vi "cfcAPDtraj.vi"(0 "file path (use dialog)":path, 1 "Save Trajectory?":bool, 2 "Trajectory length (s)":dbl=5.0 format="%#_13g", 3 "FRET Refnum":refnum<vi>, 4 "Stop Refnum":refnum<vi>, 5 "error in (no error)":errorcluster) -> (6 "FRET Traj":cluster{i32, i32}(graph), 8 "error out":errorcluster)   [LabVIEW 2015]
uses:
  <vilib>/DAQmx/write.llb/DAQmx Write (Digital Bool 1Line 1Point).vi
  <vilib>/DAQmx/read.llb/DAQmx Read (Counter 1D U32 1Chan NSamp).vi
  <vilib>/DAQmx/create/channels.llb/DAQmx Create Channel (CI-Count Edges).vi
  <vilib>/DAQmx/configure/timing.llb/DAQmx Timing (Sample Clock).vi
  <vilib>/DAQmx/create/channels.llb/DAQmx Create Channel (CO-Pulse Generation-Time).vi
  <vilib>/DAQmx/configure/trigger.llb/DAQmx Start Trigger (Digital Edge).vi
  <vilib>/DAQmx/create/channels.llb/DAQmx Create Channel (DO-Digital Output).vi
  <vilib>/DAQmx/miscellaneous.llb/DAQmx Fill In Error Info.vi
  <resource>/objmgr/daqmx.rc
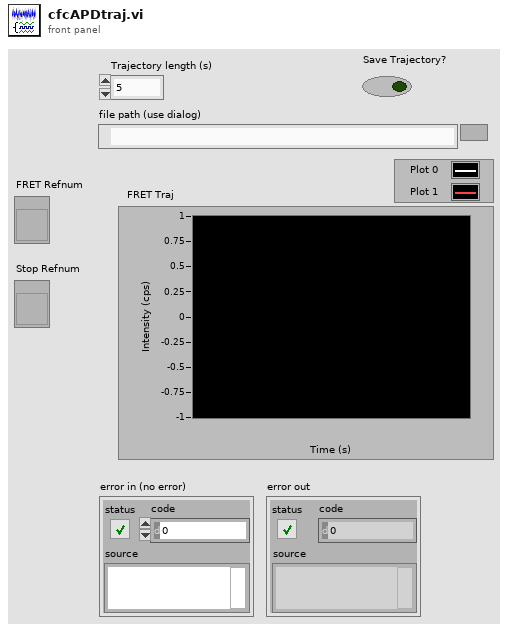
[diagram p1: front panel]
types:
  T1 = enum16{"big-endian, network order", "native, host order", "little-endian"}
  T2 = enum16{"open", "replace", "create", "open or create", "replace or create", "replace or create with confirmation"}
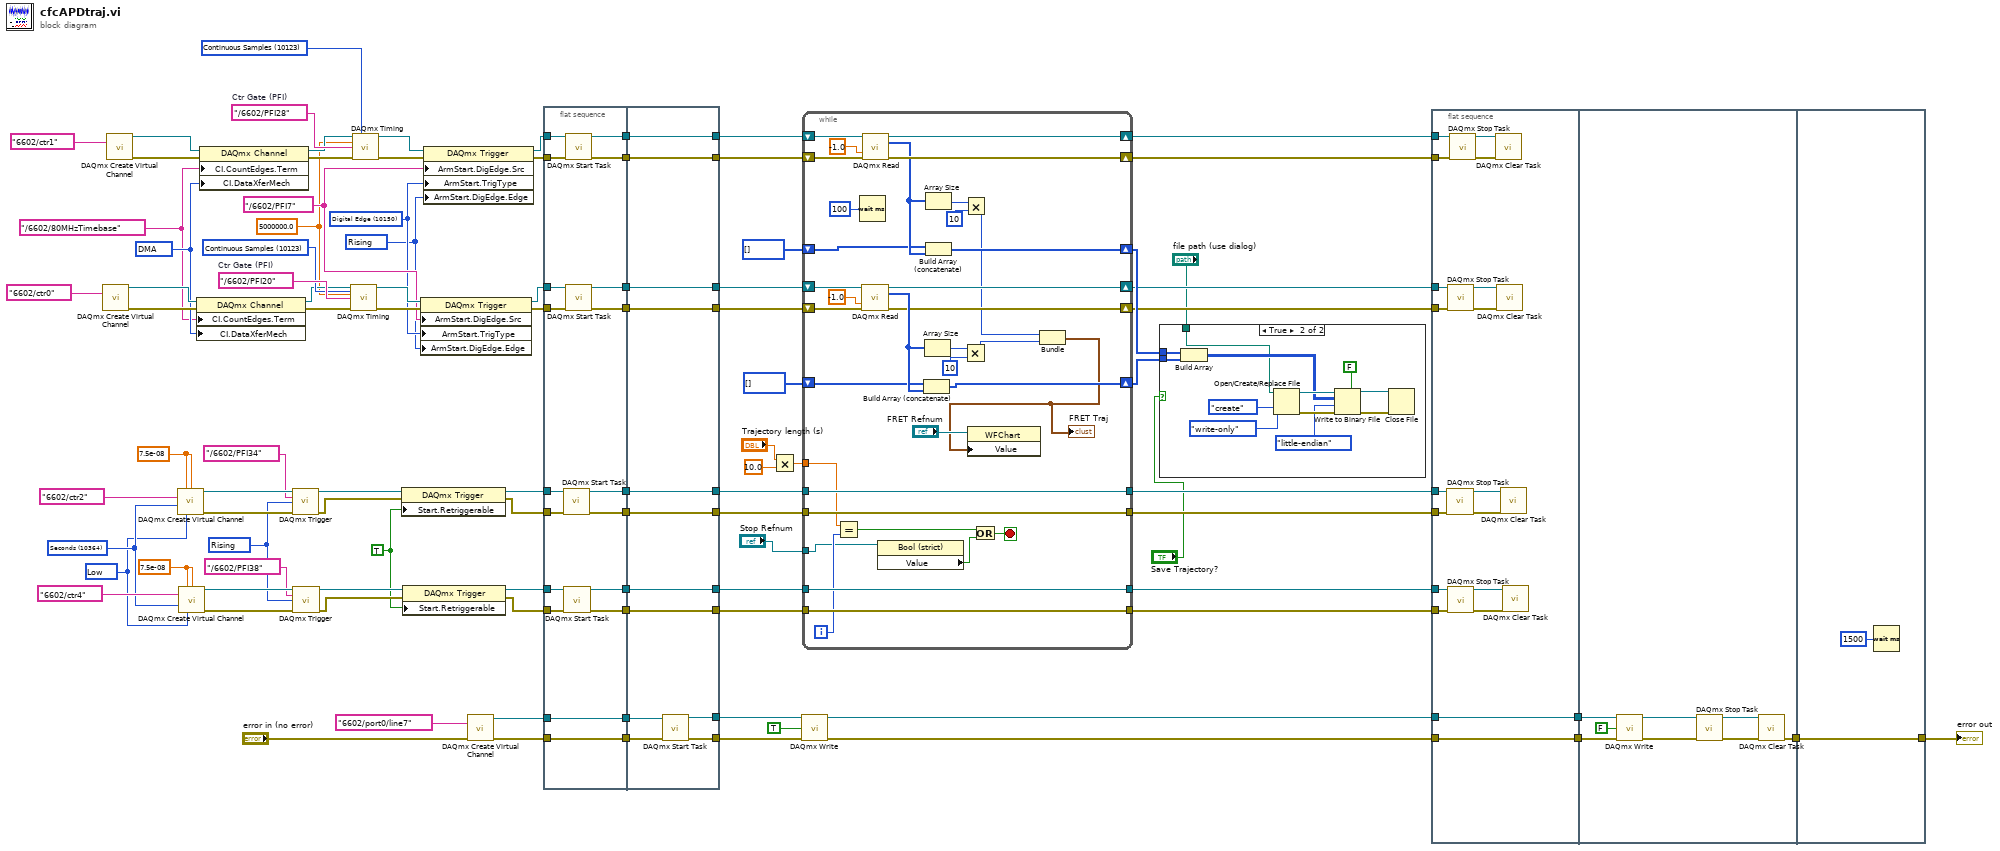
[diagram p0: block diagram]
diagram:
  w50 = 7.5e-08 ("high time")
  w73 = tag "/6602/PFI20"  # Ctr Gate (PFI)
  w68 = 10123 items=["Finite Samples"=10178, "Continuous Samples"=10123, "Hardware Timed Single Point"=12522] ("sample mode")
  w74 = 7.5e-08 ("high time")
  w42 = 10214 items=["High"=10192, "Low"=10214] ("idle state")
  w43 = 10364 items=["Seconds"=10364] ("units")
  w44 = 10280 items=["Rising"=10280, "Falling"=10171] ("edge")
  w11 = TRUE ("Start.Retriggerable")
  w49 = 10054 items=["DMA"=10054, "Interrupts"=10204, "Programmed I/O"=10264, "USB Bulk"=12590] ("CI.DataXferMech")
  w63 = tag "/6602/PFI7" ("ArmStart.DigEdge.Src")
  w61 = 10280 items=["Rising"=10280, "Falling"=10171] ("ArmStart.DigEdge.Edge")
  w62 = 10150 items=["Digital Edge"=10150, "None"=10230] ("ArmStart.TrigType")
  w99 = tag "/6602/PFI28"  # Ctr Gate (PFI)
  w93 = 10123 items=["Finite Samples"=10178, "Continuous Samples"=10123, "Hardware Timed Single Point"=12522] ("sample mode")
  w10 = 5000000.0 ("rate")
  w48 = tag "/6602/80MHzTimebase" ("CI.CountEdges.Term")
  n1 = call-poly <vilib>:"DAQmx Create Virtual Channel.vi"("counter"=tag "6602/ctr0") -> ("task out"=w71:refnum<k21>, "error out"=w70:errorcluster)  [unwired: 13 in]
  n2 = call-poly <vilib>:"DAQmx Create Virtual Channel.vi"("counter"=tag "6602/ctr1") -> ("task out"=w97:refnum<k21>, "error out"=w96:errorcluster)  [unwired: 13 in]
  n3 = call-poly <vilib>:"DAQmx Create Virtual Channel.vi"("high time"=w74, "low time"=w74, "counter"=tag "6602/ctr2", "units"=w43, "idle state"=w42) -> ("task out"=w82:refnum<k21>, "error out"=w79:errorcluster)  [unwired: 9 in]
  n4 = call-poly <vilib>:"DAQmx Create Virtual Channel.vi"("high time"=w50, "low time"=w50, "counter"=tag "6602/ctr4", "units"=w43, "idle state"=w42) -> ("task out"=w58:refnum<k21>, "error out"=w55:errorcluster)  [unwired: 9 in]
  n5 = property class="DAQmx Channel"(reference=w71, error in=w70, "CI.CountEdges.Term"=w48, "CI.DataXferMech"=w49) -> (reference out=w60:refnum<k21>, error out=w69:errorcluster)
  n6 = property class="DAQmx Channel"(reference=w97, error in=w96, "CI.CountEdges.Term"=w48, "CI.DataXferMech"=w49) -> (reference out=w94:refnum<k21>, error out=w95:errorcluster)
  n7 = call-poly <vilib>:"DAQmx Trigger.vi"("task/channels in"=w82, "source"=tag "/6602/PFI34", "edge"=w44, "error in"=w79) -> ("task out"=w81:refnum<k21>, "error out"=w78:errorcluster)  [unwired: 10 in]
  n8 = call-poly <vilib>:"DAQmx Trigger.vi"("task/channels in"=w58, "source"=tag "/6602/PFI38", "edge"=w44, "error in"=w55) -> ("task out"=w57:refnum<k21>, "error out"=w54:errorcluster)  [unwired: 10 in]
  n9 = call-poly <vilib>:"DAQmx Timing.vi"("task/channels in"=w60, "sample mode"=w68, "rate"=w10, "source"=w73, "error in"=w69) -> ("task out"=w67:refnum<k21>, "error out"=w64:errorcluster)  [unwired: 9 in]
  n10 = call-poly <vilib>:"DAQmx Timing.vi"("task/channels in"=w94, "sample mode"=w93, "rate"=w10, "source"=w99, "error in"=w95) -> ("task out"=w91:refnum<k21>, "error out"=w84:errorcluster)  [unwired: 9 in]
  n11 = property class="DAQmx Trigger"(reference=w81, error in=w78, "Start.Retriggerable"=w11) -> (reference out=w80:refnum<k21>, error out=w77:errorcluster)
  n12 = property class="DAQmx Trigger"(reference=w57, error in=w54, "Start.Retriggerable"=w11) -> (reference out=w56:refnum<k21>, error out=w53:errorcluster)
  n13 = property class="DAQmx Trigger"(reference=w67, error in=w64, "ArmStart.DigEdge.Src"=w63, "ArmStart.TrigType"=w62, "ArmStart.DigEdge.Edge"=w61) -> (reference out=w66:refnum<k21>, error out=w65:errorcluster)
  n14 = property class="DAQmx Trigger"(reference=w91, error in=w84, "ArmStart.DigEdge.Src"=w63, "ArmStart.TrigType"=w62, "ArmStart.DigEdge.Edge"=w61) -> (reference out=w90:refnum<k21>, error out=w88:errorcluster)
  n15 = call-poly <vilib>:"DAQmx Create Virtual Channel.vi"("lines"=tag "6602/port0/line7", "error in"="error in (no error)") -> ("task out"=w41:refnum<k21>, "error out"=w40:errorcluster)  [unwired: 12 in]
  n16 = flat-sequence {
    tunnel: w90 -> [w116]
    tunnel: w88 -> [w115]
    tunnel: w80 -> [w113]
    tunnel: w77 -> [w111]
    tunnel: w66 -> [w109]
    tunnel: w65 -> [w108]
    tunnel: w56 -> [w107]
    tunnel: w53 -> [w105]
    tunnel: w41 -> [w103]
    tunnel: w40 -> [w102]
    tunnel: [w117] -> w37
    tunnel: [w114] -> w36
    tunnel: [w112] -> w35
    tunnel: [w110] -> w34
    tunnel: [w106] -> w33
    tunnel: [w104] -> w32
    tunnel: [w103] -> w31
    tunnel: [w102] -> w30
    tunnel: [w101] -> w29
    tunnel: [w100] -> w28
    tunnel: [w122] -> w38
    tunnel: [w123] -> w39
    tunnel: [w124] -> w20
    tunnel: [w125] -> w21
    tunnel: [w126] -> w22
    tunnel: [w127] -> w23
    tunnel: [w128] -> w87
    tunnel: [w129] -> w92
    tunnel: w37 -> [w129]
    tunnel: w36 -> [w128]
    tunnel: w35 -> [w127]
    tunnel: w34 -> [w126]
    tunnel: w33 -> [w125]
    tunnel: w32 -> [w124]
    tunnel: w31 -> [w121]
    tunnel: w30 -> [w119]
    tunnel: w29 -> [w123]
    tunnel: w28 -> [w122]
    tunnel: [w120] -> w27
    tunnel: [w118] -> w26
    frame #0 {
      n17 = call <vilib>:"DAQmx Start Task.vi"("task/channels in"=w113, "error in"=w111) -> ("task out"=w112:refnum<k21>, "error out"=w110:errorcluster)  [unwired: 12 in]
      n18 = call <vilib>:"DAQmx Start Task.vi"("task/channels in"=w107, "error in"=w105) -> ("task out"=w106:refnum<k21>, "error out"=w104:errorcluster)  [unwired: 12 in]
      n19 = call <vilib>:"DAQmx Start Task.vi"("task/channels in"=w116, "error in"=w115) -> ("task out"=w114:refnum<k21>, "error out"=w117:errorcluster)  [unwired: 12 in]
      n20 = call <vilib>:"DAQmx Start Task.vi"("task/channels in"=w109, "error in"=w108) -> ("task out"=w101:refnum<k21>, "error out"=w100:errorcluster)  [unwired: 12 in]
    }
    frame #1 {
      n21 = call <vilib>:"DAQmx Start Task.vi"("task/channels in"=w121, "error in"=w119) -> ("task out"=w120:refnum<k21>, "error out"=w118:errorcluster)  [unwired: 12 in]
    }
  }
  n22 = Multiply(x="Trajectory length (s)", y=10.0) -> (x*y=w4:dbl)
  n23 = call-poly <vilib>:"DAQmx Write.vi"("task/channels in"=w27, "data"=TRUE ("Shutter"), "error in"=w26) -> ("task out"=w15:refnum<k21>, "error out"=w14:errorcluster)  [unwired: 10 in, 1 out]
  n24 = while {
    shift-right: [w161] -> w85
    shift-left: w92 -> [w164]
    shift-right: [w162] -> w86
    shift-left: w87 -> [w163]
    shift-right: [w154] -> w46
    shift-left: u32[] [] -> [w155]
    shift-right: [w148] -> w45
    shift-left: u32[] [] -> [w149]
    shift-right: [w144] -> w25
    shift-left: w39 -> [w147]
    shift-right: [w145] -> w24
    shift-left: w38 -> [w146]
    tunnel: w23 -> [w143]
    tunnel: [w143] -> w19
    tunnel: w22 -> [w142]
    tunnel: [w142] -> w18
    tunnel: w21 -> [w141]
    tunnel: w20 -> [w140]
    tunnel: [w141] -> w17
    tunnel: [w140] -> w16
    tunnel: w4 -> [w135]
    tunnel: "Stop Refnum" -> [w132]
    i -> [w134]
    stop <- w130 stop-if-true
    n25 = Equal?(x=w135, y=w134) -> (x = y?=w133:bool)
    n26 = Wait (ms)(milliseconds to wait=u32 100) -> ()  [unwired: 1 out]
    n27 = call-poly <vilib>:"DAQmx Read.vi"("task/channels in"=w147, "timeout"=-1.0, "error in"=w146) -> ("task out"=w144:refnum<k21>, "data"=w150:u32[], "error out"=w145:errorcluster)  [unwired: 10 in]
    n28 = call-poly <vilib>:"DAQmx Read.vi"("task/channels in"=w163, "timeout"=-1.0, "error in"=w164) -> ("task out"=w162:refnum<k21>, "data"=w156:u32[], "error out"=w161:errorcluster)  [unwired: 10 in]
    n29 = property class="Bool (strict)"(reference=w132) -> ("Value"=w131:bool)  [unwired: 1 in, 2 out]
    n30 = Build Array (concatenate)(w149, w150) -> (w148:u32[])
    n31 = Array Size(array=w150) -> (size(s)=w153:i32)
    n32 = Array Size(array=w156) -> (size(s)=w160:i32)
    n33 = Build Array (concatenate)(w155, w156) -> (w154:u32[])
    n34 = Multiply(x=w153, y=10) -> (x*y=w138:i32)
    n35 = Multiply(x=w160, y=10) -> (x*y=w139:i32)
    n36 = Or(x=w133, y=w131) -> (x .or. y?=w130:bool)
    n37 = Bundle(w139, w138) -> (w136:cluster{i32, i32})  [unwired: 1 in]
    "FRET Traj" <- w136
    n38 = property class="WFChart"(reference="FRET Refnum", "Value"=w136) -> ()  [unwired: 1 in, 2 out]
  }
  n39 = case shown="True" "Save Trajectory?" {
    tunnel: w46 -> [_ w168]
    tunnel: w45 -> [_ w167]
    tunnel: "file path (use dialog)" -> [_ w165]
    frame False {
    }
    frame True {
      n40 = Build Array(w168, w167) -> (w166:u32[][])
      n41 = Open/Create/Replace File(file path (use dialog)=w165, operation (0:open)=T2."create", access (0:read/write)=enum16{"read/write", "read-only", "write-only"}."write-only") -> (refnum out=w173:refnum<file>, error out=w174:errorcluster)  [unwired: 3 in, 1 out]
      n42 = Write to Binary File(file (use dialog)=w173, data=w166, error in=w174, 5:FALSE ("prepend array or string size? (T)"), 9:T1."little-endian" ("byte order (0:big-endian, network order)")) -> (refnum out=w170:refnum<file>, error out=w171:errorcluster)  [unwired: 1 in, 1 out]
      n43 = Close File(refnum=w170, error in=w171) -> ()  [unwired: 2 out]
    }
  }
  n44 = flat-sequence {
    tunnel: w86 -> [w192]
    tunnel: w85 -> [w191]
    tunnel: w25 -> [w184]
    tunnel: w24 -> [w183]
    tunnel: w19 -> [w182]
    tunnel: w18 -> [w181]
    tunnel: w17 -> [w180]
    tunnel: w16 -> [w179]
    tunnel: w15 -> [w178]
    tunnel: w14 -> [w177]
    tunnel: [w178] -> w13
    tunnel: [w177] -> w12
    tunnel: w13 -> [w197]
    tunnel: w12 -> [w196]
    tunnel: [w195] -> w2
    tunnel: [w204] -> w1
    tunnel: w2 -> [w204]
    frame #0 {
      n45 = call <vilib>:"DAQmx Stop Task.vi"("task/channels in"=w182, "error in"=w181) -> ("task out"=w190:refnum<k21>, "error out"=w189:errorcluster)  [unwired: 12 in]
      n46 = call <vilib>:"DAQmx Stop Task.vi"("task/channels in"=w184, "error in"=w183) -> ("task out"=w185:refnum<k21>, "error out"=w186:errorcluster)  [unwired: 12 in]
      n47 = call <vilib>:"DAQmx Stop Task.vi"("task/channels in"=w180, "error in"=w179) -> ("task out"=w188:refnum<k21>, "error out"=w187:errorcluster)  [unwired: 12 in]
      n48 = call <vilib>:"DAQmx Stop Task.vi"("task/channels in"=w192, "error in"=w191) -> ("task out"=w193:refnum<k21>, "error out"=w194:errorcluster)  [unwired: 12 in]
      n49 = call <vilib>:"DAQmx Clear Task.vi"("task in"=w193, "error in"=w194) -> ()  [unwired: 13 in, 1 out]
      n50 = call <vilib>:"DAQmx Clear Task.vi"("task in"=w185, "error in"=w186) -> ()  [unwired: 13 in, 1 out]
      n51 = call <vilib>:"DAQmx Clear Task.vi"("task in"=w190, "error in"=w189) -> ()  [unwired: 13 in, 1 out]
      n52 = call <vilib>:"DAQmx Clear Task.vi"("task in"=w188, "error in"=w187) -> ()  [unwired: 13 in, 1 out]
    }
    frame #1 {
      n53 = call-poly <vilib>:"DAQmx Write.vi"("task/channels in"=w197, "data"=FALSE, "error in"=w196) -> ("task out"=w201:refnum<k21>, "error out"=w200:errorcluster)  [unwired: 10 in, 1 out]
      n54 = call <vilib>:"DAQmx Stop Task.vi"("task/channels in"=w201, "error in"=w200) -> ("task out"=w198:refnum<k21>, "error out"=w199:errorcluster)  [unwired: 12 in]
      n55 = call <vilib>:"DAQmx Clear Task.vi"("task in"=w198, "error in"=w199) -> ("error out"=w195:errorcluster)  [unwired: 13 in]
    }
    frame #2 {
      n56 = Wait (ms)(milliseconds to wait=u32 1500) -> ()  [unwired: 1 out]
    }
  }
  "error out" <- w1
